vi "海流计数据上传20240522.vi"() -> (3 "发送的信息":string)   [LabVIEW 2016, in "数据传输系统.lvlib"]
panel:
  out "层数 2":string
  out "层数参数位置 2":i32
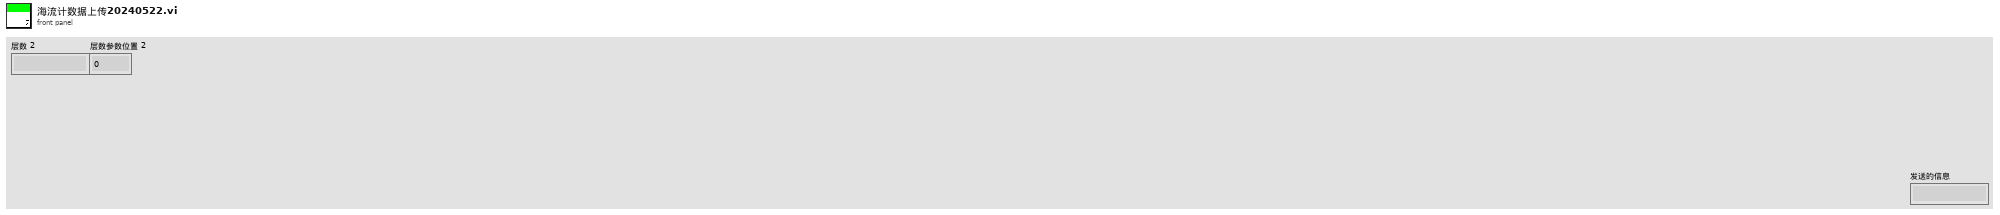
[diagram p1: front panel]
types:
  T1 = cluster{"CODMn":string, "CODCr":string, "DO":string, "铜":string, "PH":string, "氨氮":string, "比电导率":string, "水温":string, "COD":string, "浊度":string, "总氮":string, "总磷":string, "叶绿素a":string, "藻密度":string, "水位":string, "流速":string, "方向":string, "瞬时流量":string, "累积流量":string, "正累积流量":string, "负累积流量":string, "亚硝酸盐":string, "硫化物":string, "ORP":string, "铅":string, "镉":string, "锌":string, "镍":string, "锰":string, "汞":string, "气温":string, "气压":string, "风速":string, "风向":string, "空气温度":string, "相对湿度":string, "分钟雨量":string, "小时雨量":string, "日雨量":string, "累积雨量":string, "盐度":string, "磷酸盐":string, "硝氮":string, "氟化物":string, "挥发酚":string, "氯化物":string, "蓝绿藻":string, "余氯":string, "综合生物毒性":string, "艏向":string, "横摇":string, "纵摇":string, "分层标志":string, "层状态1":string, "层状态2":string, "水平平均流速":string, "流向":string, "北向流速分量":string, "东向流速分量":string, "垂直流速分量":string, "最大波高":string, "最大波周期":string, "1/10波高":string, "1/10波周期":string, "有效波高":string, "有效波周期":string, "平均波高":string, "平均波周期":string, "波向":string, "波个数":string, "水深":string}
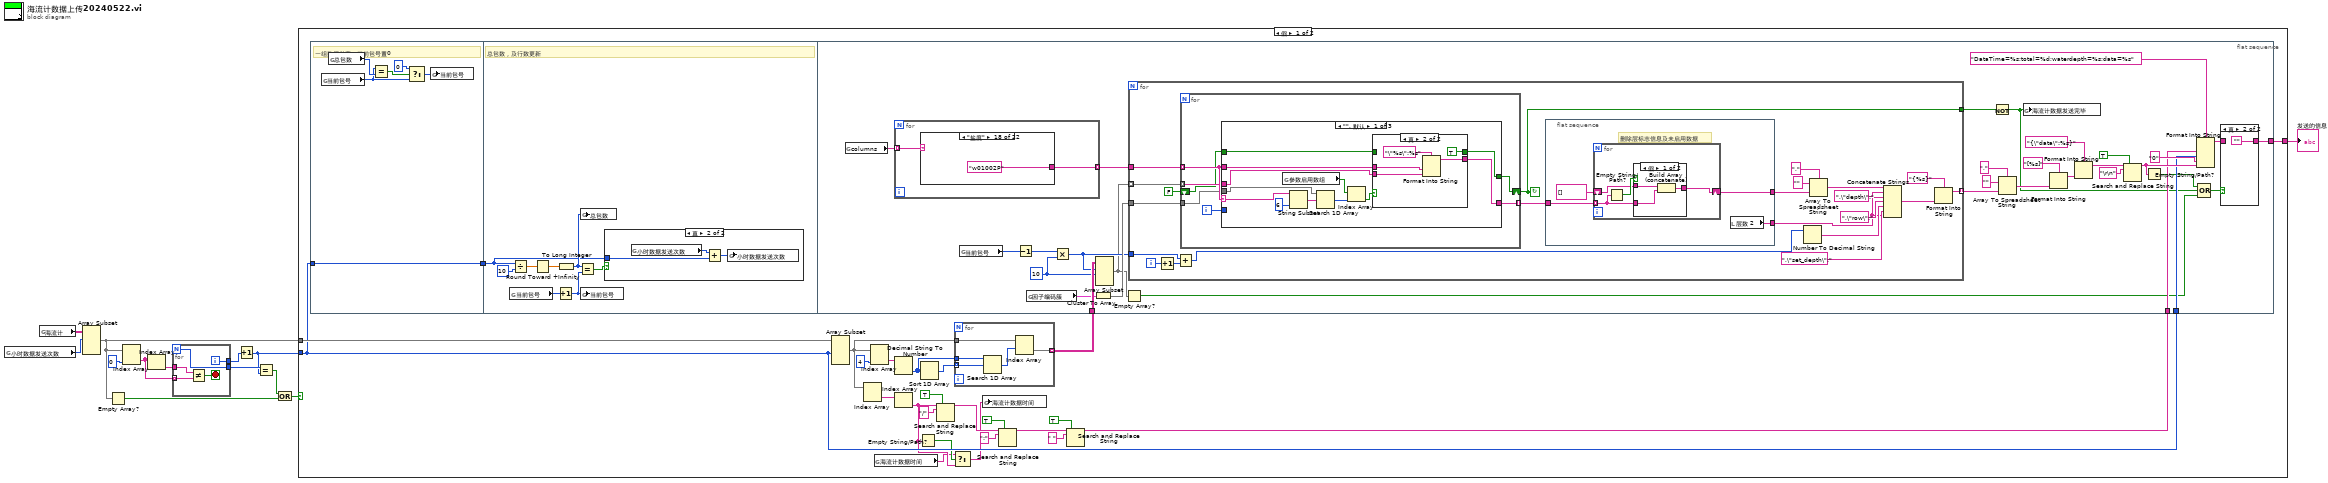
[diagram p0: block diagram]
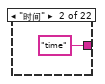
[diagram p5: hidden frame]
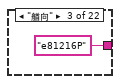
[diagram p6: hidden frame]
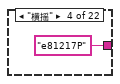
[diagram p7: hidden frame]
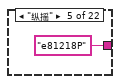
[diagram p8: hidden frame]
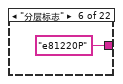
[diagram p9: hidden frame]
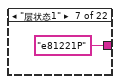
[diagram p10: hidden frame]
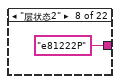
[diagram p11: hidden frame]
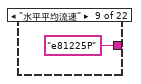
[diagram p12: hidden frame]
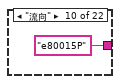
[diagram p13: hidden frame]
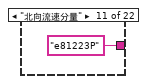
[diagram p14: hidden frame]
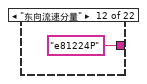
[diagram p15: hidden frame]
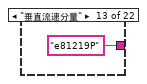
[diagram p16: hidden frame]
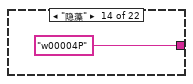
[diagram p17: hidden frame]
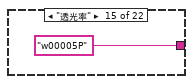
[diagram p18: hidden frame]
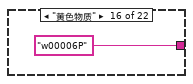
[diagram p19: hidden frame]
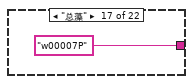
[diagram p20: hidden frame]
diagram:
  n1 = global read "全局 小时数据发送次数.vi" "小时数据发送次数"() -> (w13:i32)
  n2 = global read "全局 所有参数.vi" "海流计"() -> (w1:string[][])
  n3 = Array Subset(array=w1, index (row)=w13) -> (w4:string[][])  [unwired: 3 in]
  n4 = Empty Array?(array=w4) -> (empty?=w6:bool)
  n5 = Index Array(array=w4, index (col)=0 ("禁用的索引 (列)")) -> (element=w11:string[])  [unwired: 1 in]
  n6 = Index Array(array=w11) -> (element=w10:string)  [unwired: 1 in]
  n7 = for {
    N -> [w14]
    tunnel: w11 -> [w17] mode=indexing
    tunnel: w10 -> [w18]
    tunnel: [w15] -> w9
    tunnel: [w14] -> w8
    i -> [w15]
    stop <- w16 stop-if-true
    n8 = Not Equal?(x=w18, y=w17) -> (x != y?=w16:bool)
  }
  n9 = Increment(x=w9) -> (x+1=w7:i32)
  n10 = Equal?(x=w8, y=w7) -> (x = y?=w5:bool)
  n11 = Or(x=w5, y=w6) -> (x .or. y?=w3:bool)
  n12 = case shown="假" w3 {
    tunnel: w7 -> [w35 _]
    tunnel: w4 -> [w41 _]
    tunnel: [w19 _] -> w2
    frame False {
      n13 = flat-sequence {
        tunnel: w35 -> [w48]
        tunnel: [w48] -> w42
        tunnel: w42 -> [w54]
        tunnel: w37 -> [w96]
        tunnel: w35 -> [w74]
        tunnel: w20 -> [w73]
        tunnel: [w67] -> w19
        frame #0 {
          # "一组数据发完，当前包号置0"
          n14 = global read "全局 数据数组大小.vi" "当前包号"() -> (w51:i32)
          n15 = global read "全局 数据数组大小.vi" "总包数"() -> (w53:i32)
          n16 = Equal?(x=w51, y=w53) -> (x = y?=w52:bool)
          n17 = Select(t=0, s=w52, f=w51) -> (s? t:f=w49:i32)
          n18 = global write "全局 数据数组大小.vi" "当前包号"(w49) -> ()
        }
        frame #1 {
          # "总包数，及行数更新"
          n19 = global read "全局 数据数组大小.vi" "当前包号"() -> (w58:i32)
          n20 = Divide(x=w54, y=10) -> (x/y=w60:dbl)
          n21 = Round Toward +Infinity(x=w60) -> (ceil(x): smallest int >= x=w61:dbl)
          n22 = To Long Integer(number=w61) -> (32bit integer=w57:i32)
          n23 = Increment(x=w58) -> (x+1=w56:i32)
          n24 = Equal?(x=w57, y=w56) -> (x = y?=w55:bool)
          n25 = global write "全局 数据数组大小.vi" "总包数"(w57) -> ()
          n26 = global write "全局 数据数组大小.vi" "当前包号"(w56) -> ()
          n27 = case shown="真" w55 {
            tunnel: w54 -> [_ w63]
            frame False {
            }
            frame True {
              n28 = global read "全局 小时数据发送次数.vi" "小时数据发送次数"() -> (w64:i32)
              n29 = Add(x=w64, y=w63) -> (x+y=w62:i32)
              n30 = global write "全局 小时数据发送次数.vi" "小时数据发送次数"(w62) -> ()
            }
          }
        }
        frame #2 {
          w93 = 10 ("长度")
          n31 = global read "全局 所有参数.vi" "columns"() -> (w90:string[])
          n32 = for {
            tunnel: w90 -> [w100] mode=indexing
            tunnel: [w99] -> w89 mode=indexing
            n33 = case shown="\"盐度\"" w100 {
              tunnel: [_ "time" ("元素") "e81216P" "e81217P" "e81218P" "e81220P" "e81221P" "e81222P" "e81225P" "e80015P" "e81223P" "e81224P" "e81219P" "w00004P" "w00005P" "w00006P" "w00007P" "w01002P" "w01022P" "w81024P" "w81025P" "w81023P"] -> w99
              frame "", Default {
              }
              frame "时间" {
              }
              frame "艏向" {
              }
              frame "横摇" {
              }
              frame "纵摇" {
              }
              frame "分层标志" {
              }
              frame "层状态1" {
              }
              frame "层状态2" {
              }
              frame "水平平均流速" {
              }
              frame "流向" {
              }
              frame "北向流速分量" {
              }
              frame "东向流速分量" {
              }
              frame "垂直流速分量" {
              }
              frame "隐藻" {
              }
              frame "透光率" {
              }
              frame "黄色物质" {
              }
              frame "总藻" {
              }
              frame "盐度" {
              }
              frame "蓝绿藻" {
              }
              frame "Fv/Fm" {
              }
              frame "PAR" {
              }
              frame "GPP" {
              }
            }
          }
          n34 = global read "全局 数据数组大小.vi" "当前包号"() -> (w95:i32)
          n35 = Decrement(x=w95) -> (x-1=w94:i32)
          n36 = global read "断电保存全局.vi" "因子编码簇"() -> (w92:T1)
          n37 = Multiply(x=w94, y=w93) -> (x*y=w88:i32)
          n38 = Cluster To Array(cluster=w92) -> (array=w91:string[])
          n39 = Array Subset(array=w96, index (row)=w88, length (row)=w93) -> (w66:string[][])  [unwired: 2 in]
          n40 = Empty Array?(array=w66) -> (empty?=w65:bool)
          n41 = for {
            tunnel: w66 -> [w142] mode=indexing
            tunnel: w89 -> [w143]
            tunnel: [w138] -> w75 mode=indexing
            tunnel: w91 -> [w125]
            tunnel: [w123] -> w72
            tunnel: w88 -> [w122]
            i -> [w137]
            stop <- w123 continue-if-true
            n42 = Increment(x=w137) -> (x+1=w129:i32)
            n43 = Add(x=w122, y=w129) -> (x+y=w130:i32)
            n44 = for {
              tunnel: w143 -> [w161] mode=indexing
              tunnel: w142 -> [w160] mode=indexing
              tunnel: [w162] -> w128 mode=indexing
              tunnel: w125 -> [w158]
              shift-right: [w156] -> w123
              shift-left: FALSE -> [w157]
              i -> [w159]
              n45 = case shown="\"\", 默认" w161 {
                selector: w161 -> [w166 _ _]
                tunnel: [w174 "" w195] -> w162
                tunnel: w161 -> [w173 w186 w194]
                tunnel: w160 -> [w172 w185 w190]
                tunnel: w159 -> [_ w184 _]
                tunnel: w158 -> [w171 _ _]
                tunnel: w157 -> [w167 w182 w188]
                tunnel: [w168 w182 w188] -> w156
                frame "", Default {
                  n46 = global read "断电保存全局.vi" "参数启用数组"() -> (w170:bool[])
                  n47 = String Subset(string=w166, length (rest)=6 ("长度（剩余）")) -> (substring=w164:string)  [unwired: 1 in]
                  n48 = Search 1D Array(1D array=w171, element=w164) -> (index of element=w169:i32)  [unwired: 1 in]
                  n49 = Index Array(array=w170, index=w169) -> (element=w163:bool)
                  n50 = case shown="真" w163 {
                    tunnel: ["" w180] -> w174
                    tunnel: w173 -> [_ w179]
                    tunnel: w172 -> [_ w178]
                    tunnel: [w175 TRUE] -> w168
                    tunnel: w167 -> [w175 _]
                    frame False {
                    }
                    frame True {
                      n51 = Format Into String(format string="\"%s\":%s" ("格式字符串"), w179, w178) -> (resulting string=w180:string)  [unwired: 2 in, 1 out]
                    }
                  }
                }
                frame "e81220P" {
                  n52 = Format Into String(format string="\"%s\":%s" ("格式字符串"), w186, w185) -> ()  [unwired: 2 in, 2 out]
                  "层数 2" <- w185
                  "层数参数位置 2" <- w184
                }
                frame "time" {
                  n53 = Search and Replace String(replace all?=TRUE ("替换全部？(F)"), input string=w190, search string="/" ("搜索字符串"), replace string="-" ("替换字符串(\"\")")) -> (result string=w189:string)  [unwired: 4 in, 3 out]
                  n54 = Format Into String(format string="\"%s\":\"%s\"" ("格式字符串"), w194, w189) -> (resulting string=w195:string)  [unwired: 2 in, 1 out]
                }
              }
            }
            n55 = flat-sequence {
              tunnel: w128 -> [w146]
              tunnel: [w147] -> w127
              tunnel: [w144] -> w126
              frame #0 {
                # "删除层标志信息及未启用数据"
                n56 = for {
                  tunnel: w146 -> [w148] mode=indexing
                  shift-right: [w149] -> w144
                  shift-left: string[] [] -> [w150]
                  n57 = Empty String/Path?(string/path=w148) -> (empty?=w151:bool)
                  n58 = case shown="假" w151 {
                    tunnel: [w152 w155] -> w149
                    tunnel: w150 -> [w154 w155]
                    tunnel: w148 -> [w153 _]
                    frame False {
                      n59 = Build Array (concatenate)(w154, w153) -> (w152:string[])
                    }
                    frame True {
                    }
                  }
                }
                n60 = local read "层数 2"() -> (w147:string)
              }
            }
            n61 = Number To Decimal String(number=w130) -> (decimal integer string=w134:string)  [unwired: 1 in]
            n62 = Array To Spreadsheet String(delimiter (Tab)="," ("分隔符(Tab)"), array=w126, 3:"" ("格式字符串")) -> (spreadsheet string=w132:string)
            n63 = Concatenate Strings(w132, ",\"depth\":", w127, ",\"row\":", w134, ",\"set_depth\":", w127) -> (w131:string)
            n64 = Format Into String(format string="{%s}" ("格式字符串"), w131) -> (resulting string=w138:string)  [unwired: 2 in, 1 out]
          }
          n65 = Not(x=w72) -> (.not. x?=w70:bool)
          n66 = Array To Spreadsheet String(delimiter (Tab)="," ("分隔符(Tab)"), array=w75, 3:"" ("格式字符串")) -> (spreadsheet string=w82:string)
          n67 = global write "全局 数据数组大小.vi" "海流计数据发送完毕"(w70) -> ()
          n68 = Format Into String(format string="[%s]" ("格式字符串"), w82) -> (resulting string=w83:string)  [unwired: 2 in, 1 out]
          n69 = Format Into String(format string="{\"data\":%s}" ("格式字符串"), w83) -> (resulting string=w79:string)  [unwired: 2 in, 1 out]
          n70 = Search and Replace String(replace all?=TRUE ("替换全部？(F)"), input string=w79, search string="\r\n") -> (result string=w77:string)  [unwired: 5 in, 3 out]
          n71 = Empty String/Path?(string/path=w77) -> (empty?=w71:bool)
          n72 = Format Into String(format string="DataTime=%s;total=%d;waterdepth=%s;data=%s", w73, w74, "0" ("输入 3"), w77) -> (resulting string=w68:string)  [unwired: 2 in, 1 out]
          n73 = Compound Arithmetic op=OR ("复合运算")(w71, w70, w65) -> (w69:bool)
          n74 = case shown="真" w69 {
            tunnel: [w97 ""] -> w67
            tunnel: w68 -> [w97 _]
            frame False {
            }
            frame True {
            }
          }
        }
      }
      n75 = Array Subset(array=w41, length (row)=w35) -> (w21:string[][])  [unwired: 3 in]
      n76 = Index Array(array=w21) -> (element=w34:string[])  [unwired: 2 in]
      n77 = Index Array(array=w21, index (col)=4 ("禁用的索引 (列)")) -> (element=w40:string[])  [unwired: 1 in]
      n78 = global read "全局 水样时间.vi" "海流计数据时间"() -> (w23:string)
      n79 = Decimal String To Number(string=w40) -> (number=w39:i32[])  [unwired: 2 in, 1 out]
      n80 = Index Array(array=w34) -> (element=w24:string)  [unwired: 1 in]
      n81 = Empty String/Path?(string/path=w24) -> (empty?=w25:bool)
      n82 = Sort 1D Array(array=w39) -> (sorted array=w38:i32[])
      n83 = Search and Replace String(replace all?=TRUE ("替换全部？(F)"), input string=w24, search string="/" ("替换字符串(\"\")")) -> (result string=w29:string)  [unwired: 5 in, 3 out]
      n84 = Select(t=w23, s=w25, f=w24) -> (s? t:f=w22:string)
      n85 = for {
        tunnel: w39 -> [w47]
        tunnel: w38 -> [w46] mode=indexing
        tunnel: w21 -> [w45]
        tunnel: [w43] -> w37 mode=indexing
        n86 = Search 1D Array(1D array=w47, element=w46) -> (index of element=w44:i32)  [unwired: 1 in]
        n87 = Index Array(array=w45, index (row)=w44) -> (element=w43:string[])  [unwired: 1 in]
      }
      n88 = global write "全局 水样时间.vi" "海流计数据时间"(w22) -> ()
      n89 = Search and Replace String(replace all?=TRUE ("替换全部？(F)"), input string=w29, search string=":" ("替换字符串(\"\")")) -> (result string=w26:string)  [unwired: 5 in, 3 out]
      n90 = Search and Replace String(replace all?=TRUE ("替换全部？(F)"), input string=w26, search string=" " ("替换字符串(\"\")")) -> (result string=w20:string)  [unwired: 5 in, 3 out]
    }
    frame True {
    }
  }
  "发送的信息" <- w2
